vi "Normalize Coordinates.vi"(6 "Score":dbl, 8 "Center":cluster{"X":dbl, "Y":dbl}, 9 "Distance":dbl, 10 "Bounding box":T3, 11 "Image in":T1) -> (1 "Results":T2 {"Score" format="%#_3g"; "Pixels"."Rectangle"."Numeric 5" format="%#_3g"; "Pixels"."Rectangle"."Numeric 3" format="%#_3g"; "Pixels"."Rectangle"."Numeric 2" format="%#_3g"; "Pixels"."Rectangle"."Numeric" format="%#_3g"; "Normalized"."Rectangle"."Numeric 5" format="%#_2g"; "Normalized"."Rectangle"."Numeric 3" format="%#_2g"; "Normalized"."Rectangle"."Numeric 2" format="%#_2g"; "Normalized"."Rectangle"."Numeric" format="%#_2g"; "Normalized"."Center"."?" format="%#_3g"; "Normalized"."Center"."?" format="%#_3g"; "Distance (ft)" format="%#_3g"}, 3 "Image out":T1)   [LabVIEW 2025]
doc: "Normalize the rectangle and center so that they range from -1 to 1, left to right and bottom to top. This helps with producing joystick coordinates for driving the robot and makes the code better at handling resolution changes of the camera."
uses:
  <vilib>/vision/Image Controls.llb/IMAQ Image.ctl
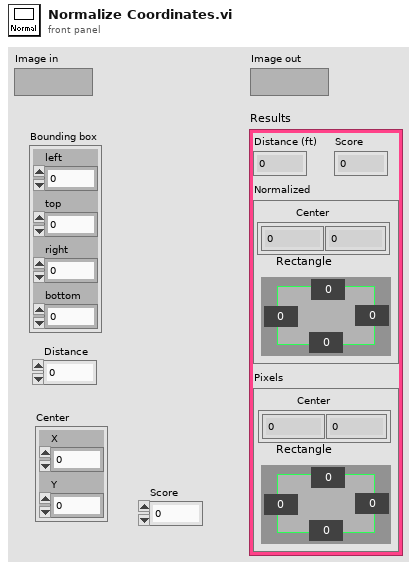
[diagram p1: front panel]
types:
  T1 = typedef "IMAQ Image.ctl" = refnum<image>
  T2 = cluster{"Distance (ft)":dbl, "Score":dbl, "Normalized":cluster{"Center":cluster{dbl, dbl}, "Rectangle":cluster{"Numeric":dbl, "Numeric 2":dbl, "Numeric 3":dbl, "Numeric 5":dbl}}, "Pixels":cluster{"Center":cluster{dbl, dbl}, "Rectangle":cluster{"Numeric":dbl, "Numeric 2":dbl, "Numeric 3":dbl, "Numeric 5":dbl}}}
  T3 = cluster{"left":dbl, "top":dbl, "right":dbl, "bottom":dbl}
  T4 = cluster{"X Resolution":i32, i32, "X Resolution":i32, i32}
  T5 = cluster{"Center":cluster{"X":dbl, "Y":dbl}, "Bounding box":cluster{"left":dbl, "top":dbl, "right":dbl, "bottom":dbl}}
  T6 = cluster{cluster{dbl, dbl}, cluster{dbl, dbl, dbl, dbl}}
  T7 = cluster{"Distance":dbl, "Score":dbl, cluster{cluster{dbl, dbl}, cluster{dbl, dbl, dbl, dbl}}, cluster{"Center":cluster{"X":dbl, "Y":dbl}, "Bounding box":cluster{"left":dbl, "top":dbl, "right":dbl, "bottom":dbl}}}
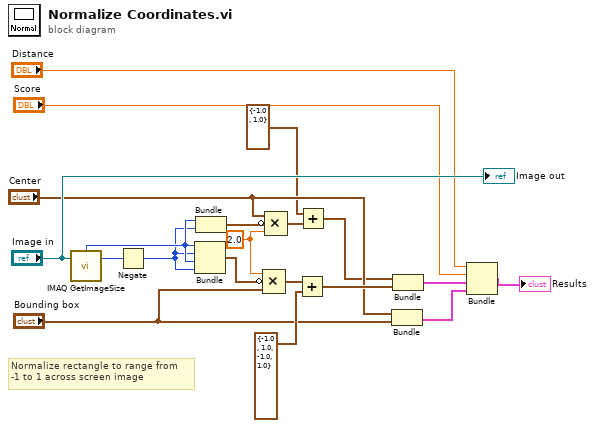
[diagram p0: block diagram]
diagram:
  w7 = 2.0
  # "Normalize rectangle to range from\n-1 to 1 across screen image"
  n1 = call "IMAQ GetImageSize"("Image"="Image in") -> ("Y Resolution"=w20:i32, "X Resolution"=w10:i32)  [unwired: 3 in, 1 out]
  n2 = Negate(x=w20) -> (-x=w9:i32)
  n3 = Bundle("X Resolution"=w10, w9, "X Resolution"=w10, w9) -> (w18:T4)  [unwired: 1 in]
  n4 = Bundle("X Resolution"=w10, w9) -> (w8:cluster{"X Resolution":i32, i32})  [unwired: 1 in]
  n5 = Compound Arithmetic op=MULTIPLY(w7, invert w18, "Bounding box") -> (w17:cluster{dbl, dbl, dbl, dbl})
  n6 = Compound Arithmetic op=MULTIPLY("Center", invert w8, w7) -> (w5:cluster{dbl, dbl})
  n7 = Add(x=w17, y=cluster{dbl, dbl, dbl, dbl} {-1.0, 1.0, -1.0, 1.0}) -> (x+y=w16:cluster{dbl, dbl, dbl, dbl})
  n8 = Add(x=cluster{dbl, dbl} {-1.0, 1.0} ("y"), y=w5) -> (x+y=w4:cluster{dbl, dbl})
  n9 = Bundle("Center"="Center", "Bounding box"="Bounding box") -> (w11:T5)  [unwired: 1 in]
  n10 = Bundle(w4, w16) -> (w14:T6)  [unwired: 1 in]
  n11 = Bundle("Distance"="Distance", "Score"="Score", w14, w11) -> (→"Results":T7)  [unwired: 1 in]
  "Image out" <- "Image in"
